vi "Status Created Events.vi"(11 "Base Queue in":refnum<class "Base Queue.lvclass">) -> (0 "Created Event Count":i32, 1 "Created Event Aliases":string[](array[string]), 2 "Created Event Exist?":bool, 3 "Base Queue out":refnum<class "Base Queue.lvclass">)   [LabVIEW 2021, in "jettl.lvlib" / "Base Queue.lvlib" / "Base Queue.lvclass"]
uses:
  Base Queue.lvclass
  C:/git/jettl/jettl/jettl/jettl/jettl.lvclass
  Base Queue.lvclass/Base Queue.ctl
  Addresses/Addresses.lvlib
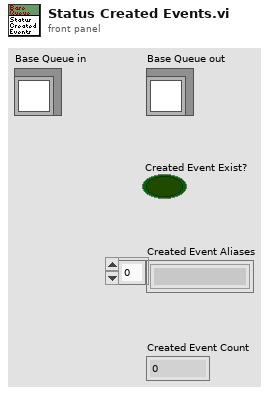
[diagram p1: front panel]
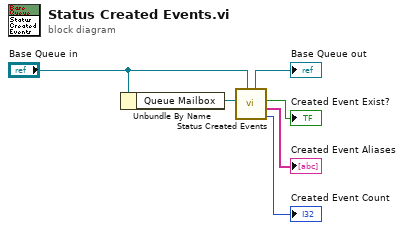
[diagram p0: block diagram]
diagram:
  n1 = Unbundle By Name("Base Queue in") -> ("Queue Mailbox"=w6:refnum<data-value>)
  n2 = call "Status Created Events.vi"("jettl in"="Base Queue in", "Queue Mailbox"=w6) -> ("Created Event Count"=→"Created Event Count":i32, "Created Event Aliases"=→"Created Event Aliases":string[], "Created Event Exist?"=→"Created Event Exist?":bool, "jettl out"=→"Base Queue out":refnum<class "Base Queue.lvclass">)  [unwired: 6 in]
